vi "setUp.vi"(8 "error in (no error)":errorcluster, 11 "reference in":refnum<class "Object Comparisons.lvclass">) -> (0 "error out":errorcluster, 3 "reference in":refnum<class "Object Comparisons.lvclass">)   [LabVIEW 2009, in "Object Comparisons.lvclass"]
doc: "setUp runs prior to the test method during test execution. Use this method to initialize any object data required by your tests."
uses:
  Object Comparisons.lvclass
  <vilib>/addons/_JKI Toolkits/VI Tester/TestCase.llb/TestCase.lvclass
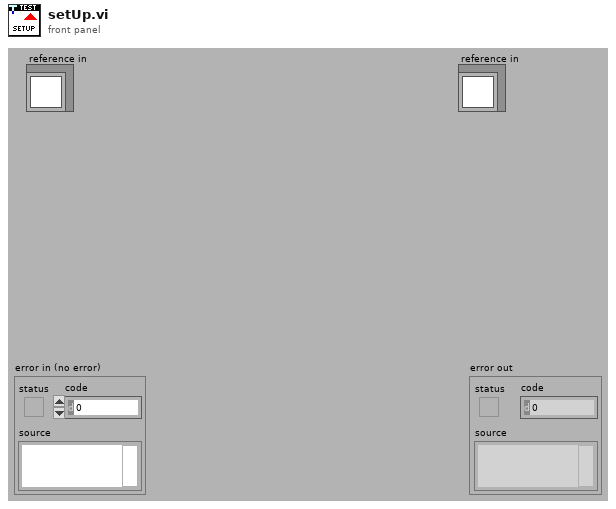
[diagram p1: front panel]
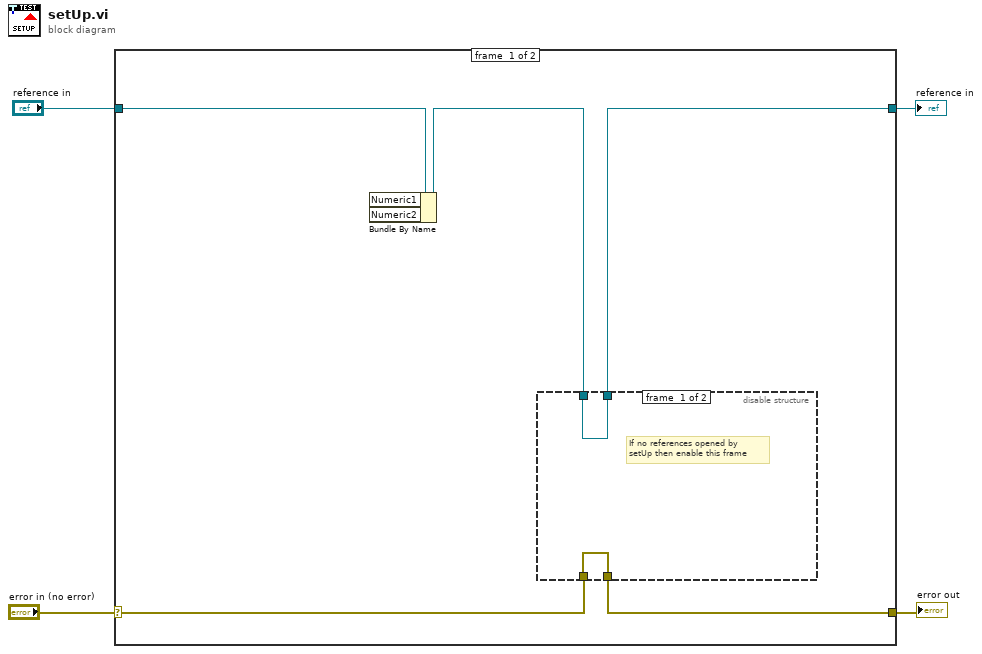
[diagram p0: block diagram]
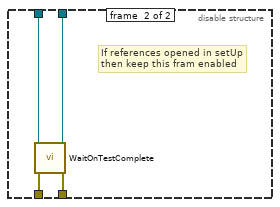
[diagram p2: hidden frame]
diagram:
  n1 = case shown="No Error" "error in (no error)" {
    selector: "error in (no error)" -> [w6 w17]
    tunnel: [w5 w17] -> w3
    tunnel: [w7 w16] -> w1
    tunnel: "reference in" -> [w9 w16]
    frame #0 {
      n2 = Bundle By Name(cluster=w9) -> (w8:refnum<class "Object Comparisons.lvclass">)  [unwired: 2 in]
      n3 = disable-structure shown="Enabled" {
        disable-tunnel: w8 -> [w11 w15]
        disable-tunnel: [w11 w14] -> w7
        disable-tunnel: w6 -> [w10 w13]
        disable-tunnel: [w10 w12] -> w5
        frame #0 {
          # "If no references opened by\nsetUp then enable this frame"
        }
        frame #1 {
          # "If references opened in setUp\nthen keep this fram enabled"
          n4 = call <vilib>:"WaitOnTestComplete.vi"("error in (no error)"=w13, "TestCase in"=w15) -> ("error out"=w12:errorcluster, "TestCase out"=w14:refnum<class "Object Comparisons.lvclass">)  [unwired: 8 in]
        }
      }
    }
    frame #1 {
    }
  }
  "error out" <- w3
  "reference in" <- w1
